vi "Set Property.vi"(8 "error in (no error)":errorcluster caption="错误输入（无错误）", 9 "Value":variant, 10 "Property Name":string, 11 "Item输入":refnum<class "Item.lvclass">) -> (0 "error out":errorcluster caption="错误输出", 3 "Item输出":refnum<class "Item.lvclass">, 4 "replaced":bool)   [LabVIEW 2013, in "Hierarchy Framework.lvlib" / "Item.lvclass"]
doc: "Sets a <B>Property Name</B> and <B>Value</B> for an item property and saves this information in the system definition file. If the <B>Property Name</B> you specify already exists, this VI overwrites the property. Wire data to the <B>Value</B> input to determine the polymorphic instance to use or manually select the instance."
uses:
  Item.lvclass
  Item.lvclass/Item.ctl
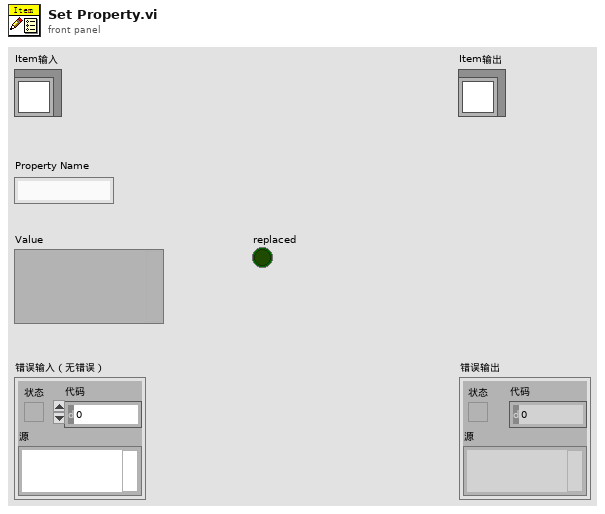
[diagram p1: front panel]
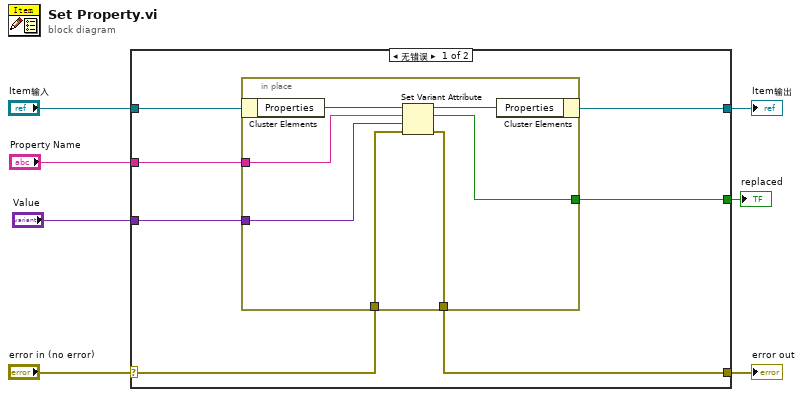
[diagram p0: block diagram]
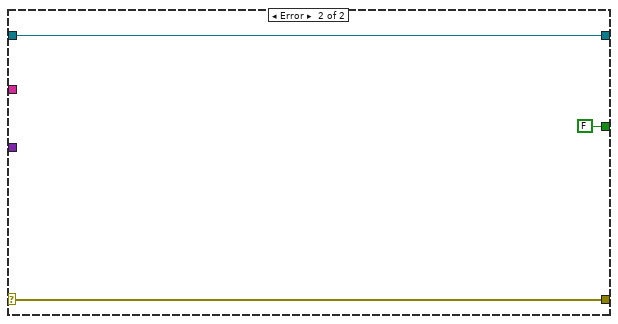
[diagram p2: hidden frame]
diagram:
  n1 = case shown="无错误" "error in (no error)" {
    selector: "error in (no error)" -> [w9 w24]
    tunnel: [w8 w24] -> w6
    tunnel: [w13 w23] -> w4
    tunnel: "Item输入" -> [w14 w23]
    tunnel: [w12 FALSE ("replaced")] -> w1
    tunnel: "Property Name" -> [w11 _]
    tunnel: "Value" -> [w10 _]
    frame No Error {
      n2 = in-place {
        in-place-border: [w19] -> w12
        in-place-border: w11 -> [w18]
        in-place-border: w10 -> [w17]
        in-place-border: w9 -> [w16]
        in-place-border: [w15] -> w8
        n3 = in-place-cluster #1(w14) -> ("Properties"=w21:variant)
        n4 = Set Variant Attribute(Variant=w21, name=w18, value=w17, error in=w16) -> (Variant out=w20:variant, replaced=w19:bool, error out=w15:errorcluster)
        n5 = in-place-cluster #1("Properties"=w20) -> (w13:refnum<class "Item.lvclass">)
      }
    }
    frame Error {
    }
  }
  "error out" <- w6
  "Item输出" <- w4
  "replaced" <- w1
